vi "InitFolderTree.vi"   [LabVIEW 2019]
doc: "This VI instantiates the FRC 4265 standard roboRIO file tree if necessary."
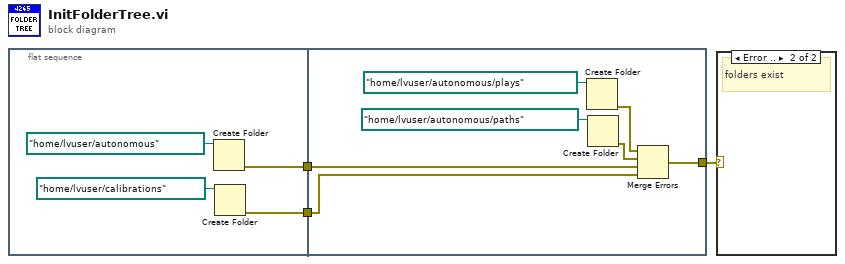
[diagram p0: block diagram]
diagram:
  n1 = flat-sequence {
    tunnel: [w6] -> w3
    tunnel: [w4] -> w2
    tunnel: w3 -> [w10]
    tunnel: [w9] -> w1
    tunnel: w2 -> [w8]
    frame #0 {
      n2 = Create Folder(path (use dialog)=path "/home/lvuser/autonomous") -> (error out=w6:errorcluster)  [unwired: 2 in, 2 out]
      n3 = Create Folder(path (use dialog)=path "/home/lvuser/calibrations") -> (error out=w4:errorcluster)  [unwired: 2 in, 2 out]
    }
    frame #1 {
      n4 = Create Folder(path (use dialog)=path "/home/lvuser/autonomous/plays") -> (error out=w12:errorcluster)  [unwired: 2 in, 2 out]
      n5 = Create Folder(path (use dialog)=path "/home/lvuser/autonomous/paths") -> (error out=w11:errorcluster)  [unwired: 2 in, 2 out]
      n6 = Merge Errors(w12, w11, w10, w8) -> (w9:errorcluster)
    }
  }
  n7 = case shown="Error .." w1 {
    frame No Error {
      # "folders created"
    }
    frame Error {
      # "folders exist"
    }
  }
